vi "insertqueur.vi"(3 "error in (no error)":errorcluster, 4 "queue":T1, 5 "VISA Session":refnum<visa-resource-name>) -> (0 "error out":errorcluster, 1 "queue out":T1)   [LabVIEW 2011]
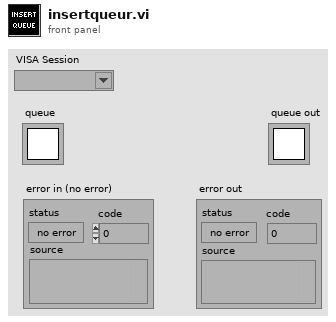
[diagram p1: front panel]
types:
  T1 = typedef "Queue RefNum" = refnum<k1>
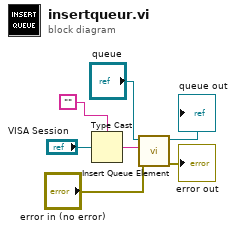
[diagram p0: block diagram]
diagram:
  n1 = Type Cast(type="", x="VISA Session") -> (*(type *) &x=w6:string)
  n2 = call <vilib>:"Insert Queue Element.vi"("error in (no error)"="error in (no error)", "queue element"=w6, "queue"="queue") -> ("error out"=→"error out":errorcluster, "queue out"=→"queue out":T1)  [unwired: 4 in, 1 out]
